vi "Host Image Acquisition Module.vi"(0 "Operation":T3=enum."Close FPGA", 11 "error in":errorcluster={"status"=FALSE, "code"=61003, "source"="niLvFpga_Run_PCIe-1473R-LX110.vi"}) -> (1 "Number of Elements to Read Cam Data":u32, 3 "Num Frames read":u32, 4 "Image":T2(plugin-control), 6 "Acq In Progress":bool, 8 "error out":errorcluster={"status"=FALSE, "code"=61003, "source"="niLvFpga_Run_PCIe-1473R-LX110.vi"}, 10 "Image Acquired":bool, 12 "Number of Elements to Write Host DMA":u32, 14 "DMA Write Timeout":bool, 15 "Frames To Acquire":u32=1)   [LabVIEW 2013]
uses:
  Host Image Acquisition Module Enum.ctl
  Acquisition Settings Cluster.ctl
  Image Acquisition Settings FG Enum.ctl
  Common/CL Configuration.ctl
  Common/CL Signal Mapping.ctl
  System Status/Status FG Enum.ctl
  Image Processing/Mask ROI FG Enum.ctl
  <vilib>/rvi/interface/common/niFpgaWaitOnOcc.vi
  Globals/Average Sector Data.vi
  <vilib>/Utility/error.llb/Error Cluster From Error Code.vi
  <vilib>/rvi/errors/niLvFpgaAdjustHostInterfaceError.vi
  <vilib>/FPGAPlugInAG/PCIe-1473R-LX110/niLvFpga_Run_PCIe-1473R-LX110.vi
  <vilib>/FPGAPlugInAG/PCIe-1473R-LX110/niLvFpga_Close_PCIe-1473R-LX110.vi
  <vilib>/rvi/interface/nirviReadWriteControl/nirviReadWriteControl.xnode
  FGs/FPGA_Reference.ctl
  FPGA Bitfiles/WBA256SectorsSim_FPGATarget.lvbitx
  <vilib>/rvi/interface/nirviMethod/nirviMethod.xnode
  FPGA/Sector/Accumulate/Sector Parameter Cluster.ctl
  <vilib>/rvi/interface/nirviCloseFPGA/nirviCloseFPGA.xnode
  Common/Timing/Timing Lib.lvlib
  NiFpgaLv.dll
  <vilib>/FPGAPlugInAG/PCIe-1473R-LX110/niLvFpga_ReadFifo_PCIe-1473R-LX110.vi
  <vilib>/rvi/errors/niLvFpgaMergeErrorWithErrorCode.vi
  <vilib>/FPGAPlugInAG/PCIe-1473R-LX110/niLvFpga_ConfigureFifo_PCIe-1473R-LX110.vi
  <vilib>/FPGAPlugInAG/PCIe-1473R-LX110/niLvFpga_StartFifo_PCIe-1473R-LX110.vi
  <vilib>/FPGAPlugInAG/PCIe-1473R-LX110/niLvFpga_Reset_PCIe-1473R-LX110.vi
panel:
  out "Actual Depth":u32=53190144
  out "Target Sim TO":bool
  out "Cam Data Timeout":bool
  out "Sector FIFO Timeout":bool
  out "Host DMA Timeout":bool
  out "Elements Remaining":u32
  out "Words per image":u32=118200
  out "DMA Words per Image":u32=118200
  out "Acquire":bool=TRUE
  in  "Acquisition Settings Cluster":T1={"Image Width"=1200, "Image Height"=788, "Frames To Acquire"=0, "Signal Mapping"=enum."Basler 10-tap", "DMA Buffer Size\n(In Images)"=64} {"Image Height" max=65535; "Image Width" max=65535 step=40}
  out "Buffer Size":u32=53190000
  out "Acq'd Frame Width":u32
  in  "Start Serial Server":bool
  out "Frames Acq'd":u32=1
  out "Acq'd Frame Height":u32
  out "Initialized":bool
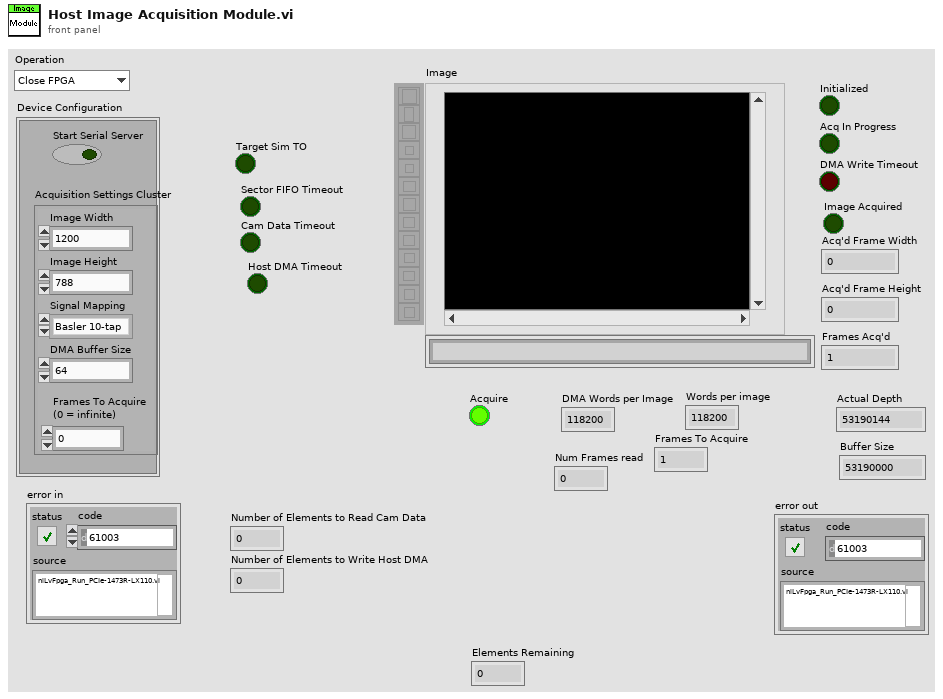
[diagram p1: front panel]
types:
  T1 = typedef "Acquisition Settings Cluster.ctl" = cluster{"Image Width":u32, "Image Height":u32, "Frames To Acquire":u32, "Signal Mapping":enum8{"Standard", "Basler 10-tap", "Vosskühler 10-tap"}, "DMA Buffer Size\n(In Images)":u32}
  T2 = typedef "IMAQ Image.ctl" = refnum<image>
  T3 = typedef "Host Image Acquisition Module Enum.ctl" = enum16{"Open FPGA", "Initialize DMA FIFO", "Load Sim Images", "Initialize Acquisition", "Update Sector Parameters", "Start Acquisition", "Aquire Image", "Read Averages", "Cancel Acquisition", "Close FPGA"}
  T4 = typedef "CL Signal Mapping.ctl" = enum8{"Standard", "Basler 10-tap", "Vosskühler 10-tap"}
  T5 = typedef "CL Configuration.ctl" = enum8{"Base", "Medium", "Full"}
  T6 = typedef "Image Acquisition Settings FG Enum.ctl" = enum16{"Read", "Write"}
  T7 = typedef "Status FG Enum.ctl" = enum16{"Reset", "Read", "Write"}
  T8 = typedef "Mask ROI FG Enum.ctl" = enum16{"Read", "Write", "Enable Background", "Disable Background"}
  T9 = enum16{"big-endian, network order", "native, host order", "little-endian"}
  T10 = typedef "FPGA_Reference.ctl" = refnum<k20>
  T11 = typedef "Mask ROI Cluster.ctl" = cluster{"left annulus":T12, "right annulus":T12, "Threshold Range":cluster{"Lower value":dbl, "Upper value":dbl}, "[Avg BG]":u8[], "Number of Sectors":u8, "Left ROI":T13, "Right ROI":T13, "Left Start Angle Duty Cycle":fxp<+,8,0>, "Left End Angle Duty Cycle":fxp<+,8,0>, "Right End Angle Duty Cycle":fxp<+,8,0>, "Right Start Angle Duty Cycle":fxp<+,8,0>, "[Sector ROIs]":T13[]}
  T12 = typedef "IMAQ Circle" = cluster{"Center X":i32, "Center Y":i32, "Inner Radius":i32, "Outer Radius":i32, "Start Angle":dbl, "End Angle":dbl}
  T13 = typedef "ROI Descriptor" = cluster{"Global Rectangle":i32[], "Contours":cluster{"ID":enum32{"External", "Internal"}, "Type":u32, "Coordinates":i32[]}[]}
  T14 = typedef "Sector Parameter Cluster.ctl" = cluster{"Start Angle":fxp<+/-,17,2>, "End Angle":fxp<+/-,17,2>, "Inner Radius":u16, "Outter Radius":u16, "Hinge X":u16, "Hinge Y":u16, "NumWingSectors":u8}
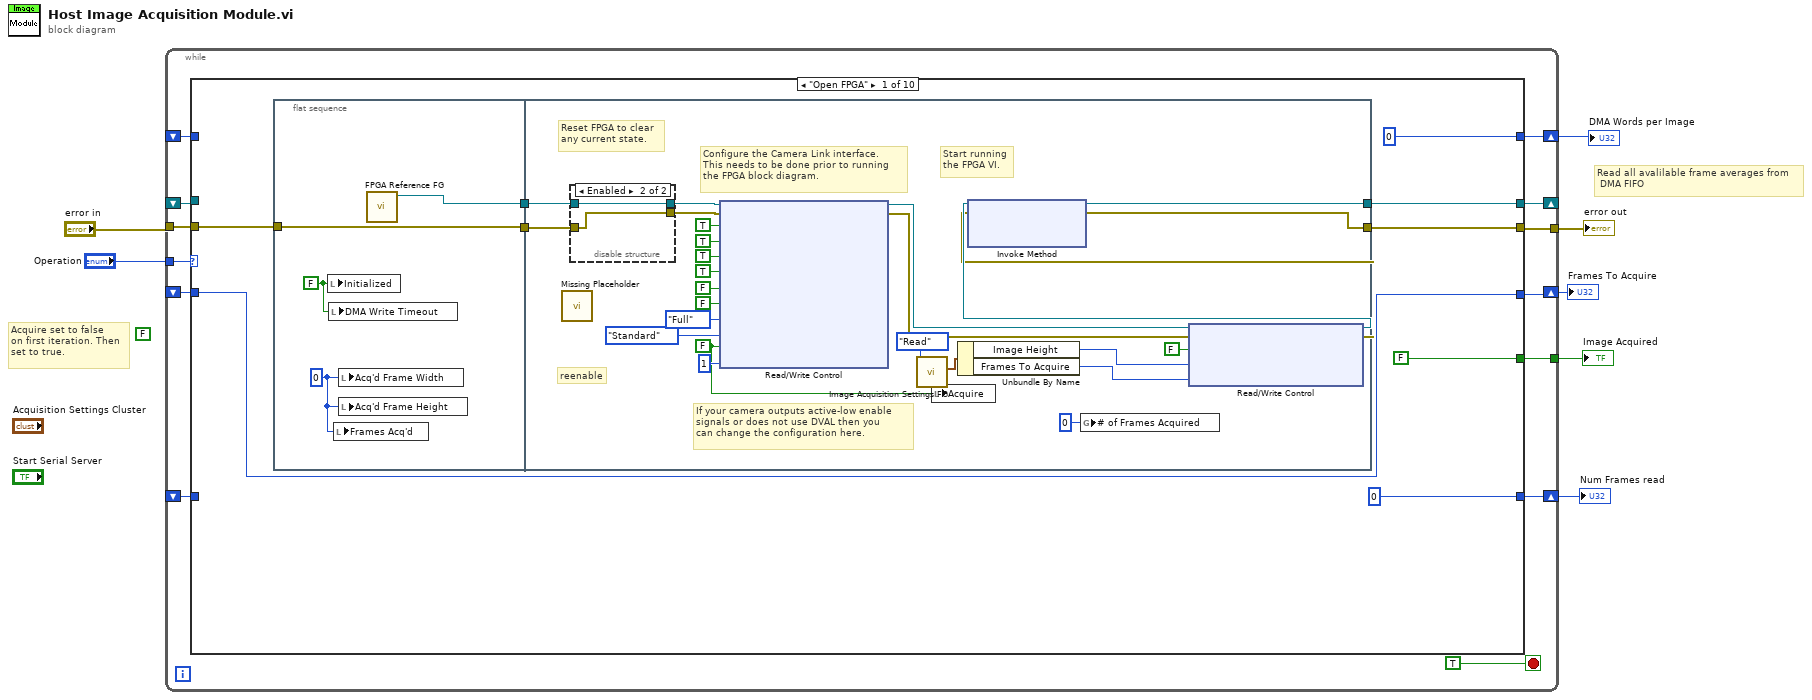
[diagram p0: block diagram]
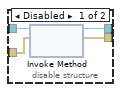
[diagram p2: hidden frame]
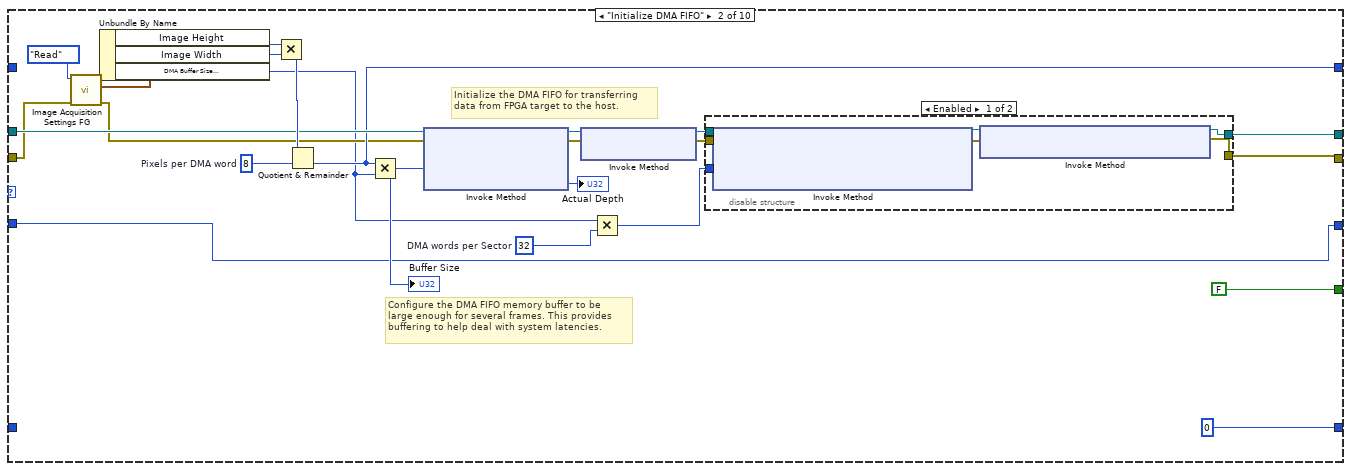
[diagram p3: hidden frame]
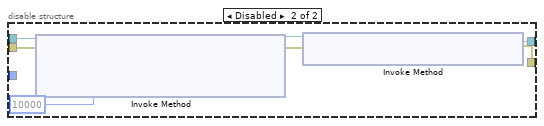
[diagram p4: hidden frame]
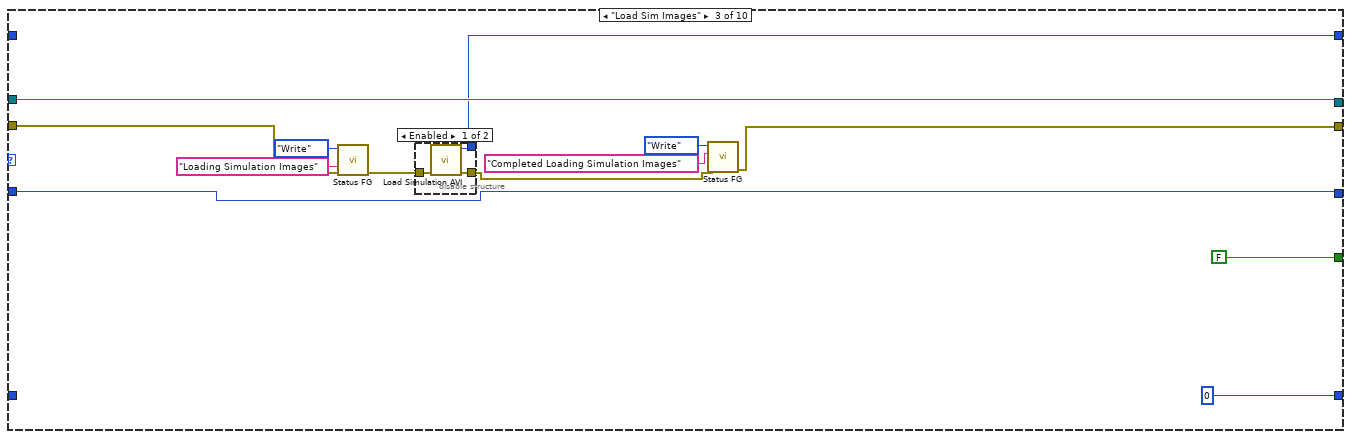
[diagram p5: hidden frame]
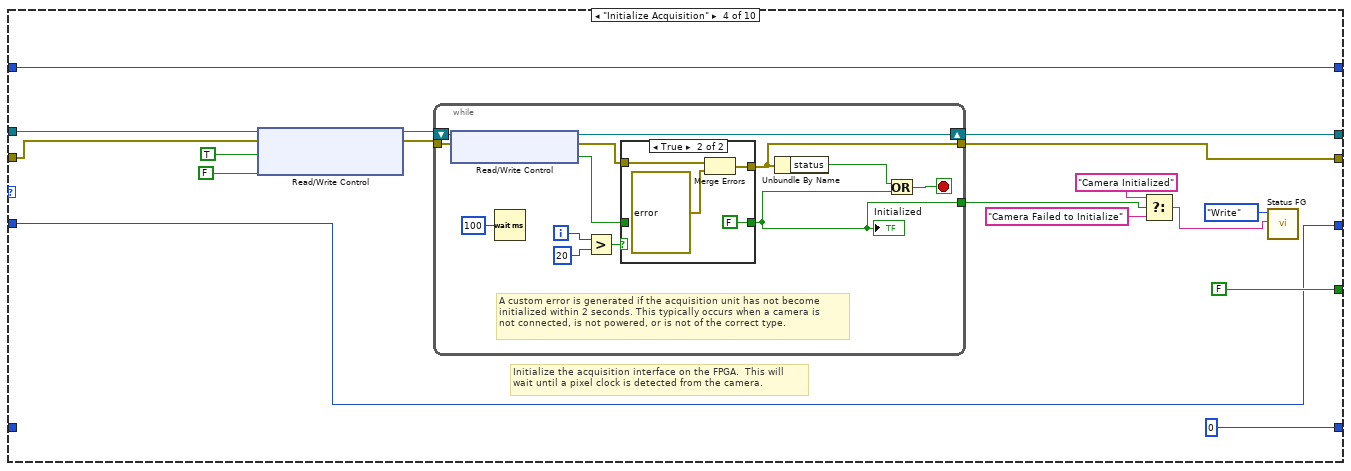
[diagram p7: hidden frame]
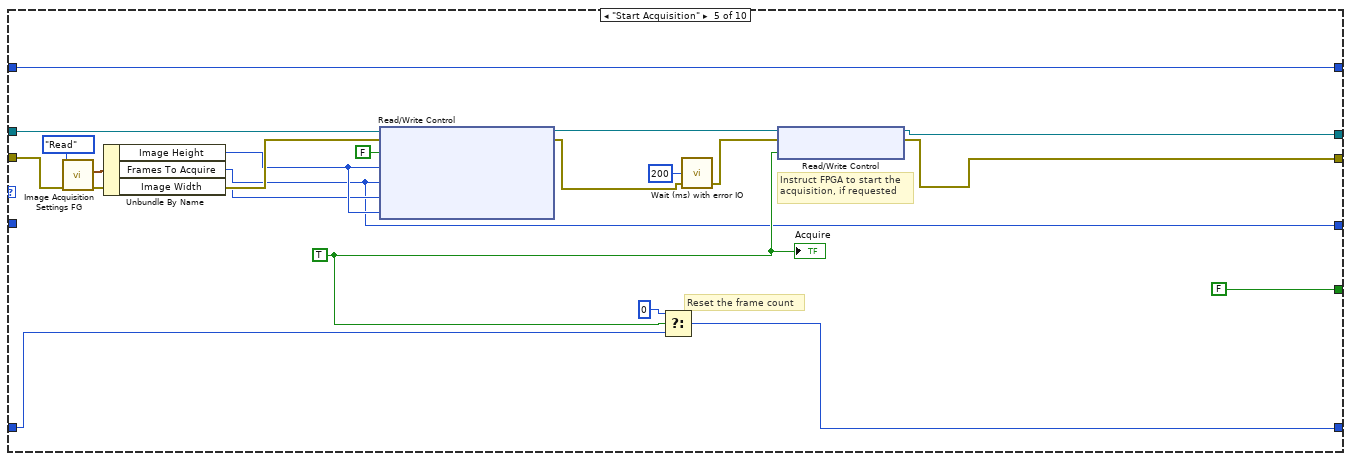
[diagram p9: hidden frame]
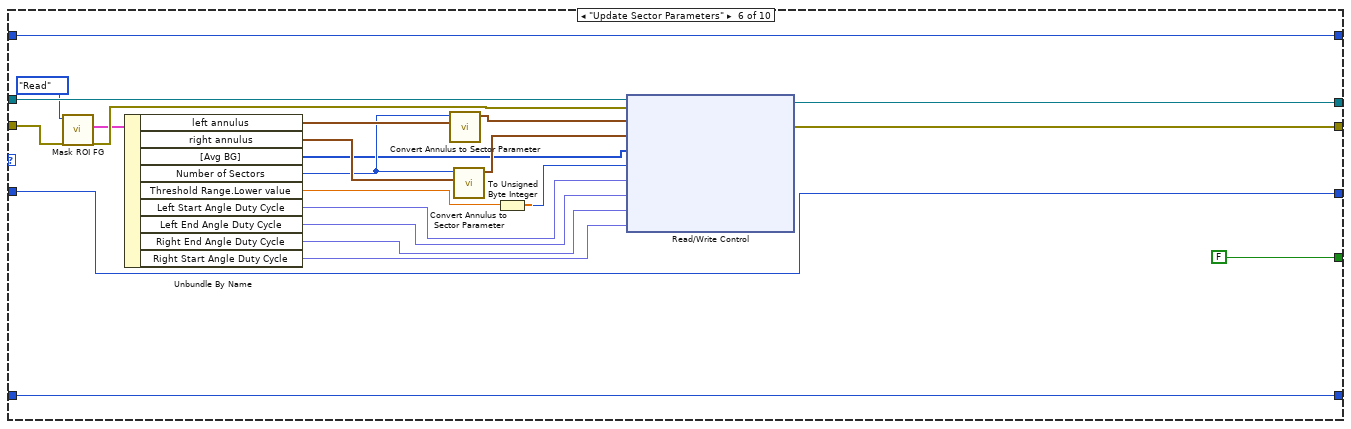
[diagram p10: hidden frame]
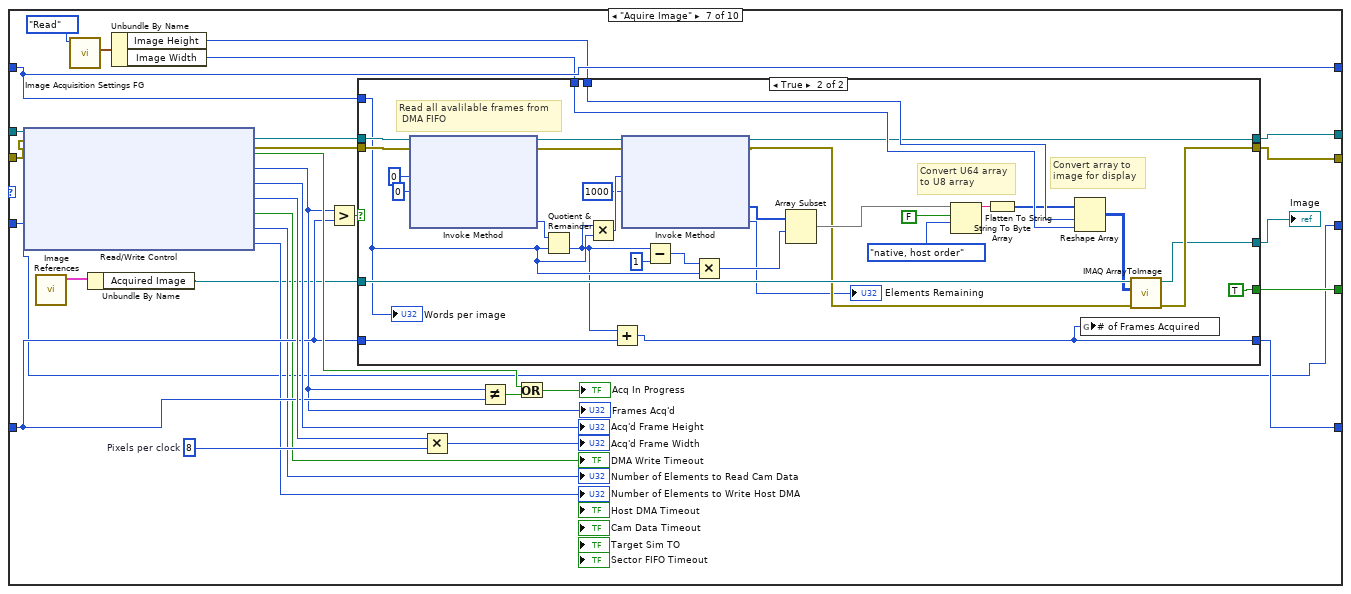
[diagram p11: hidden frame]
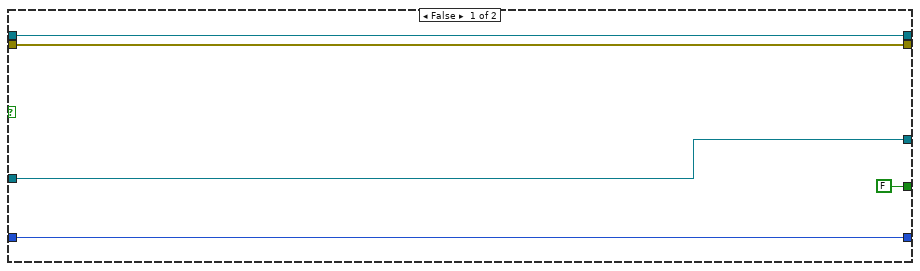
[diagram p12: hidden frame]
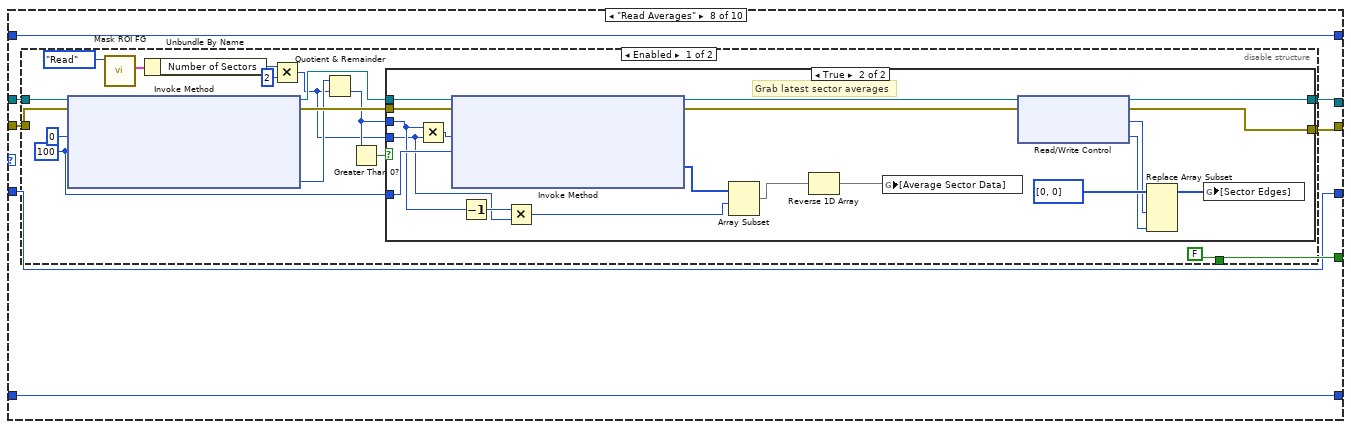
[diagram p13: hidden frame]
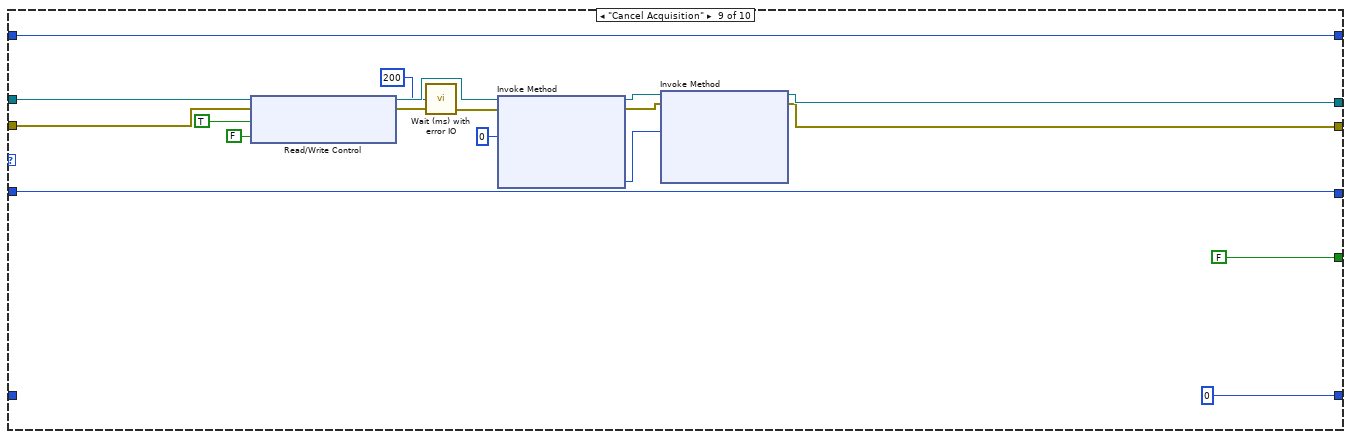
[diagram p16: hidden frame]
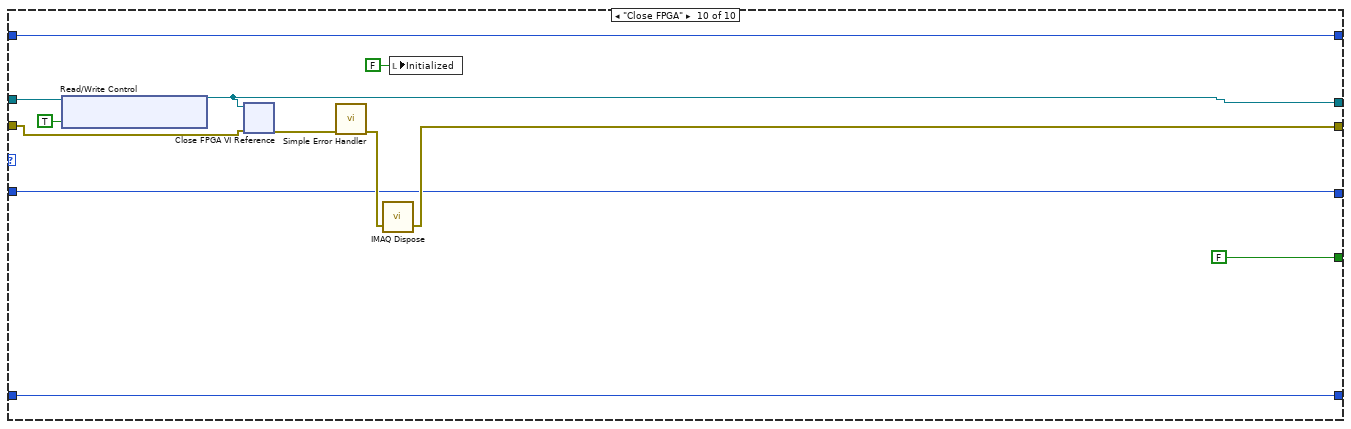
[diagram p17: hidden frame]
diagram:
  (unwired) FALSE ("Acquire")
  # "Read all avalilable frame averages from\n DMA FIFO"
  # "Acquire set to false\non first iteration. Then\nset to true."
  n1 = while {
    shift-right: [w19] -> _
    shift-left: _ -> [w15]
    tunnel: "error in" -> [w18]
    tunnel: "Operation" -> [w17]
    tunnel: [w16] -> w5
    shift-right: [w14] -> w4
    shift-left: _ -> [w13]
    shift-right: [w12] -> w3
    shift-left: _ -> [w11]
    tunnel: [w10] -> w2
    shift-right: [w9] -> w1
    shift-left: _ -> [w8]
    stop <- TRUE stop-if-true
    n2 = case shown="\"Open FPGA\"" w17 {
      tunnel: w18 -> [w29 w79 w112 w128 w172 w198 w214 w269 w331 w336]
      tunnel: [w28 w75 w115 w133 w166 w194 w229 w274 w317 w337] -> w19
      tunnel: [w27 w70 w106 w129 w165 w195 w228 w270 w316 w342] -> w16
      tunnel: w15 -> [_ w84 w115 w134 w173 w200 w230 w275 w333 w339]
      tunnel: [u32 0 w83 w114 w132 w168 w199 w223 w273 w330 w340] -> w14
      tunnel: w13 -> [_ _ _ w132 w168 w199 w223 w273 w330 w340]
      tunnel: [u32 0 u32 0 u32 0 u32 0 w169 w193 w227 w272 u32 0 w341] -> w12
      tunnel: w11 -> [_ _ _ _ w170 w193 w212 w272 _ w341]
      tunnel: [FALSE ("Image Acquired") FALSE ("Image Acquired") FALSE ("Image Acquired") FALSE ("Image Acquired") FALSE ("Image Acquired") FALSE ("Image Acquired") w208 w271 FALSE ("Image Acquired") FALSE ("Image Acquired")] -> w10
      tunnel: [w21 w66 w104 w121 w157 w178 w201 w268 w326 w334] -> w9
      tunnel: w8 -> [w21 w66 w104 w121 _ w178 w201 w268 w326 w334]
      frame "Open FPGA" {
        n3 = flat-sequence {
          tunnel: w29 -> [w30]
          tunnel: [w31] -> w26
          tunnel: [w30] -> w25
          tunnel: [w48] -> w27
          tunnel: [w49] -> w28
          tunnel: w26 -> [w52]
          tunnel: w25 -> [w50]
          frame #0 {
            w32 = u32 0 ("Acq'd Frame Width")
            w33 = FALSE ("Initialized")
            n4 = local write "Initialized"(w33) -> ()
            n5 = local write "DMA Write Timeout"(w33) -> ()
            n6 = local write "Frames Acq'd"(w32) -> ()
            n7 = local write "Acq'd Frame Width"(w32) -> ()
            n8 = local write "Acq'd Frame Height"(w32) -> ()
            n9 = call "FPGA Reference FG.vi"() -> ("FPGA VI Reference Out"=w31:T10)  [unwired: 11 in]
          }
          frame #1 {
            w46 = FALSE ("Acq Control.Acquire")
            # "reenable"
            # "If your camera outputs active-low enable\nsignals or does not use DVAL then you \ncan change the configuration here."
            # "Start running\nthe FPGA VI."
            # "Reset FPGA to clear\nany current state."
            # "Configure the Camera Link interface.\nThis needs to be done prior to running\nthe FPGA block diagram."
            n10 = call "Missing Placeholder.vi"() -> ()  [unwired: 12 in]
            n11 = disable-structure shown="Enabled" {
              disable-tunnel: [w63 w65] -> w54
              disable-tunnel: [w62 w64] -> w53
              disable-tunnel: w52 -> [w61 w65]
              disable-tunnel: w50 -> [w60 w64]
              frame Disabled {
                n12 = xnode "Invoke Method"("FPGA VI Reference In"=w61, "error in"=w60) -> ("FPGA VI Reference Out"=w63:T10, "error out"=w62:errorcluster)
              }
              frame Enabled {
              }
            }
            n13 = xnode "Read/Write Control"("FPGA VI Reference In"=w54, "error in"=w53, "CL Config.FVAL Active High"=TRUE ("IO Module Config.CL FVAL Active High"), "CL Config.LVAL Active High"=TRUE ("IO Module Config.CL LVAL Active High"), "CL Config.DVAL Active High"=TRUE ("IO Module Config.CL DVAL Active High"), "CL Config.Spare Active High"=TRUE ("IO Module Config.CL Spare Active High"), "CL Config.Line Scan"=FALSE, "Acq Control.Ignore DVAL"=FALSE ("CL Config.Line Scan"), "CL Config.Configuration"=CL_Configuration."Full", "CL Config.Signal Mapping"=CL_Signal_Mapping."Standard", "Acq Control.Acquire"=w46, "# of Frames to Average"=u8 1) -> ("FPGA VI Reference Out"=w41:T10, "error out"=w39:errorcluster)
            n14 = call "Image Acquisition Settings FG.vi"("Operation"=Image_Acquisition_Settings_FG_Enum."Read") -> ("Acquisition Settings Out"=w45:T1)  [unwired: 9 in, 1 out]
            n15 = local write "Acquire"(w46) -> ()
            n16 = Unbundle By Name(w45) -> ("Image Height"=w43:u32, "Frames To Acquire"=w37:u32)
            n17 = global write "Average Sector Data.vi" "# of Frames Acquired"(u32 0 ("# of Frames Acquired")) -> ()
            n18 = xnode "Read/Write Control"("FPGA VI Reference In"=w41, "error in"=w39, "Acq Control.Cancel Acq"=FALSE, "Acq Control.Line Scan Height"=w43, "Acq Control.Frames To Acq"=w37) -> ("FPGA VI Reference Out"=w40:T10, "error out"=w38:errorcluster)
            n19 = xnode "Invoke Method"("FPGA VI Reference In"=w40, "error in"=w38) -> ("FPGA VI Reference Out"=w49:T10, "error out"=w48:errorcluster)  [unwired: 1 in]
          }
        }
      }
      frame "Initialize DMA FIFO" {
        w69 = u32 32  # DMA words per Sector
        w86 = u32 8  # Pixels per DMA word
        # "Configure the DMA FIFO memory buffer to be\nlarge enough for several frames. This provides\nbuffering to help deal with system latencies."
        # "Initialize the DMA FIFO for transferring\ndata from FPGA target to the host."
        n20 = call "Image Acquisition Settings FG.vi"("error in (no error)"=w79, "Operation"=Image_Acquisition_Settings_FG_Enum."Read") -> ("error out"=w76:errorcluster, "Acquisition Settings Out"=w80:T1)  [unwired: 8 in]
        n21 = Unbundle By Name(w80) -> ("Image Height"=w78:u32, "Image Width"=w77:u32, "DMA Buffer Size\n(In Images)"=w68:u32)
        n22 = Multiply(x=w78, y=w77) -> (x*y=w85:u32)
        n23 = Quotient & Remainder(x=w85, y=w86) -> (floor(x/y)=w83:u32)  [unwired: 1 out]
        n24 = Multiply(x=w83, y=w68) -> (x*y=w87:u32)
        "Buffer Size" <- w87
        n25 = xnode "Invoke Method"("FPGA VI Reference In"=w84, "error in"=w76, "Requested Depth"=w87) -> ("FPGA VI Reference Out"=w89:T10, "error out"=w88:errorcluster, "Actual Depth"=→"Actual Depth":u32)
        n26 = xnode "Invoke Method"("FPGA VI Reference In"=w89, "error in"=w88) -> ("FPGA VI Reference Out"=w73:T10, "error out"=w71:errorcluster)
        n27 = Multiply(x=w68, y=w69) -> (x*y=w67:u32)
        n28 = disable-structure shown="Enabled" {
          disable-tunnel: w67 -> [w96 _]
          disable-tunnel: [w95 w103] -> w75
          disable-tunnel: w73 -> [w94 w102]
          disable-tunnel: w71 -> [w93 w101]
          disable-tunnel: [w90 w98] -> w70
          frame Enabled {
            n29 = xnode "Invoke Method"("FPGA VI Reference In"=w94, "error in"=w93, "Requested Depth"=w96) -> ("FPGA VI Reference Out"=w92:T10, "error out"=w91:errorcluster)  [unwired: 1 out]
            n30 = xnode "Invoke Method"("FPGA VI Reference In"=w92, "error in"=w91) -> ("FPGA VI Reference Out"=w95:T10, "error out"=w90:errorcluster)
          }
          frame Disabled {
            n31 = xnode "Invoke Method"("FPGA VI Reference In"=w102, "error in"=w101, "Requested Depth"=u32 10000) -> ("FPGA VI Reference Out"=w100:T10, "error out"=w99:errorcluster)  [unwired: 1 out]
            n32 = xnode "Invoke Method"("FPGA VI Reference In"=w100, "error in"=w99) -> ("FPGA VI Reference Out"=w103:T10, "error out"=w98:errorcluster)
          }
        }
      }
      frame "Load Sim Images" {
        n33 = call "Status FG.vi"("error in (no error)"=w112, "Status In"="Loading Simulation Images", "Operation"=Status_FG_Enum."Write") -> ("error out"=w111:errorcluster)  [unwired: 7 in, 1 out]
        n34 = disable-structure shown="Enabled" {
          disable-tunnel: [w119 _] -> w114
          disable-tunnel: w111 -> [w118 w120]
          disable-tunnel: [w117 w120] -> w107
          frame Enabled {
            n35 = call "Load Simulation AVI.vi"("error in (no error)"=w118) -> ("error out"=w117:errorcluster, "Words per image"=w119:u32)  [unwired: 9 in]
          }
          frame Disabled {
          }
        }
        n36 = call "Status FG.vi"("error in (no error)"=w107, "Status In"="Completed Loading Simulation Images", "Operation"=Status_FG_Enum."Write") -> ("error out"=w106:errorcluster)  [unwired: 7 in, 1 out]
      }
      frame "Initialize Acquisition" {
        # "Initialize the acquisition interface on the FPGA.  This will\nwait until a pixel clock is detected from the camera."
        n37 = xnode "Read/Write Control"("FPGA VI Reference In"=w134, "error in"=w128, "Acq Control.Initialize"=TRUE ("Arm Acquisition"), "Acq Control.Cancel Acq"=FALSE) -> ("FPGA VI Reference Out"=w137:T10, "error out"=w136:errorcluster)
        n38 = while {
          tunnel: w136 -> [w145]
          tunnel: [w147] -> w129
          shift-right: [w144] -> w133
          shift-left: w137 -> [w146]
          tunnel: [w138] -> w124
          i -> [w140]
          stop <- w150 stop-if-true
          # "A custom error is generated if the acquisition unit has not become\ninitialized within 2 seconds. This typically occurs when a camera is\nnot connected, is not powered, or is not of the correct type."
          n39 = xnode "Read/Write Control"("FPGA VI Reference In"=w146, "error in"=w145) -> ("FPGA VI Reference Out"=w144:T10, "error out"=w143:errorcluster, "Acq Status.Initialized"=w142:bool)
          n40 = Wait (ms)(milliseconds to wait=u32 100) -> ()  [unwired: 1 out]
          n41 = Greater?(x=w140, y=20) -> (0:w141:bool)
          n42 = case shown="True" w141 {
            tunnel: [w152 FALSE] -> w138
            tunnel: w142 -> [w152 _]
            tunnel: w143 -> [w151 w154]
            tunnel: [w151 w156] -> w147
            frame False {
            }
            frame True {
              n43 = Merge Errors(w154, errorcluster {"status"=TRUE, "code"=-8999, "source"="Acquisition Initialization: This error typically occurs when a camera is not properly connected, is not powered, or is not of the correct type."} ("error in")) -> (w156:errorcluster)
            }
          }
          "Initialized" <- w138
          n44 = Unbundle By Name(w147) -> ("status"=w149:bool)
          n45 = Or(x=w149, y=w138) -> (x .or. y?=w150:bool)
        }
        n46 = Select(t="Camera Initialized", s=w124, f="Camera Failed to Initialize") -> (s? t:f=w126:string)
        n47 = call "Status FG.vi"("Status In"=w126, "Operation"=Status_FG_Enum."Write") -> ()  [unwired: 8 in, 2 out]
      }
      frame "Start Acquisition" {
        w174 = TRUE ("Acquire")
        # "Reset the frame count"
        # "Instruct FPGA to start the\nacquisition, if requested"
        n48 = call "Image Acquisition Settings FG.vi"("error in (no error)"=w172, "Operation"=Image_Acquisition_Settings_FG_Enum."Read") -> ("error out"=w171:errorcluster, "Acquisition Settings Out"=w177:T1)  [unwired: 8 in]
        n49 = Unbundle By Name(w177) -> ("Image Height"=w159:u32, "Frames To Acquire"=w157:u32, "Image Width"=w158:u32)
        n50 = xnode "Read/Write Control"("FPGA VI Reference In"=w173, "error in"=w171, "Acq Control.Cancel Acq"=FALSE, "Acq Control.Line Scan Height"=w159, "Acq Control.Frames To Acq"=w157, "X Resolution"=w158, "Y Resolution"=w159) -> ("FPGA VI Reference Out"=w163:T10, "error out"=w162:errorcluster)
        n51 = Select(t=u32 0, s=w174, f=w170) -> (s? t:f=w169:u32)
        n52 = call "Wait (ms) with error IO.vi"("error in (no error)"=w162, "milliseconds to wait"=u32 200) -> ("error out"=w161:errorcluster)  [unwired: 3 in]
        n53 = xnode "Read/Write Control"("FPGA VI Reference In"=w163, "error in"=w161, "Acq Control.Acquire"=w174) -> ("FPGA VI Reference Out"=w166:T10, "error out"=w165:errorcluster)
        "Acquire" <- w174
      }
      frame "Update Sector Parameters" {
        n54 = call "Mask ROI FG.vi"("error in (no error)"=w198, "Operation"=Mask_ROI_FG_Enum."Read") -> ("error out"=w197:errorcluster, "Mask ROI Out"=w192:T11)  [unwired: 8 in]
        n55 = Unbundle By Name(w192) -> ("left annulus"=w191:T12, "right annulus"=w189:T12, "[Avg BG]"=w186:u8[], "Number of Sectors"=w188:u8, "Threshold Range.Lower value"=w184:dbl, "Left Start Angle Duty Cycle"=w182:fxp<+,8,0>, "Left End Angle Duty Cycle"=w181:fxp<+,8,0>, "Right End Angle Duty Cycle"=w180:fxp<+,8,0>, "Right Start Angle Duty Cycle"=w179:fxp<+,8,0>)
        n56 = call "Convert Annulus to Sector Parameter.vi"("Annulus"=w191, "NumWingSectors"=w188) -> ("Sector Parameter"=w190:T14)  [unwired: 9 in]
        n57 = call "Convert Annulus to Sector Parameter.vi"("Annulus"=w189, "NumWingSectors"=w188) -> ("Sector Parameter"=w187:T14)  [unwired: 9 in]
        n58 = To Unsigned Byte Integer(number=w184) -> (unsigned 8bit integer=w183:u8)
        n59 = xnode "Read/Write Control"("FPGA VI Reference In"=w200, "error in"=w197, "Sector Parameters Left"=w190, "Sector Parameters Right"=w187, "[Average BG Intensity]"=w186, "Sector Threshold"=w183, "Left Start Angle Duty Cycle"=w182, "Left End Angle Duty Cycle"=w181, "Right End Angle Duty Cycle"=w180, "Right Start Angle Duty Cycle"=w179) -> ("FPGA VI Reference Out"=w194:T10, "error out"=w195:errorcluster)
      }
      frame "Aquire Image" {
        w221 = u32 8  # Pixels per clock
        n60 = xnode "Read/Write Control"("FPGA VI Reference In"=w230, "error in"=w214) -> ("FPGA VI Reference Out"=w226:T10, "error out"=w225:errorcluster, "Acq Status.Acq In Progress"=w213:bool, "Acq Status.Frames Acq'd"=w211:u32, "Acq Status.Lines Per Frame"=→"Acq'd Frame Height":u32, "Acq Status.Clocks Per Line"=w220:u32, "Acq Status.DMA Write Timeout"=→"DMA Write Timeout":bool, "Number of Elements to Read Cam Data"=→"Number of Elements to Read Cam Data":u32, "Number of Elements to Write Host DMA"=→"Number of Elements to Write Host DMA":u32)
        "Frames Acq'd" <- w211
        n61 = call "Image References.vi"() -> ("Images"=w204:cluster{"Acquired Image":T2, "Display Image":T2})  [unwired: 10 in, 1 out]
        n62 = call "Image Acquisition Settings FG.vi"("Operation"=Image_Acquisition_Settings_FG_Enum."Read") -> ("Acquisition Settings Out"=w217:T1)  [unwired: 9 in, 1 out]
        n63 = Unbundle By Name(w204) -> ("Acquired Image"=w203:T2)
        n64 = Unbundle By Name(w217) -> ("Image Height"=w216:u32, "Image Width"=w215:u32)
        n65 = Greater?(x=w211, y=w212) -> (0:w224:bool)
        n66 = case shown="True" w224 {
          tunnel: w226 -> [w234 w259]
          tunnel: w225 -> [w233 w260]
          tunnel: w216 -> [_ w267]
          tunnel: w215 -> [_ w266]
          tunnel: w203 -> [w235 w265]
          tunnel: [w233 w264] -> w228
          tunnel: [w234 w240] -> w229
          tunnel: w212 -> [w232 w263]
          tunnel: [w232 w238] -> w227
          tunnel: w223 -> [_ w245]
          tunnel: [w235 w262] -> w202
          tunnel: [FALSE ("Image Acquired") TRUE ("Image Acquired")] -> w208
          frame False {
          }
          frame True {
            # "Convert U64 array\nto U8 array"
            # "Convert array to\nimage for display"
            # "Read all avalilable frames from\n DMA FIFO"
            n67 = xnode "Invoke Method"("FPGA VI Reference In"=w259, "error in"=w260, "Number of Elements"=u32 0, "Timeout (ms)"=0) -> ("FPGA VI Reference Out"=w256:T10, "error out"=w255:errorcluster, "Elements Remaining"=w254:u32)  [unwired: 1 out]
            n68 = Quotient & Remainder(x=w254, y=w245) -> (floor(x/y)=w236:u32)  [unwired: 1 out]
            n69 = Multiply(x=w236, y=w245) -> (x*y=w253:u32)
            n70 = Add(x=w236, y=w263) -> (x+y=w238:u32)
            n71 = xnode "Invoke Method"("FPGA VI Reference In"=w256, "error in"=w255, "Number of Elements"=w253, "Timeout (ms)"=1000) -> ("FPGA VI Reference Out"=w240:T10, "error out"=w241:errorcluster, "Data"=w244:u64[], "Elements Remaining"=→"Elements Remaining":u32)
            n72 = Subtract(x=w236, y=u32 1) -> (x-y=w246:u32)
            n73 = Multiply(x=w246, y=w245) -> (x*y=w243:u32)
            n74 = Array Subset(array=w244, index=w243) -> (w242:u64[])  [unwired: 1 in]
            n75 = Flatten To String(anything=w242, prepend array or string size? (T)=FALSE, byte order (0:big-endian, network order)=T9."native, host order") -> (data string=w248:string)  [unwired: 1 in, 2 out]
            n76 = String To Byte Array(string=w248) -> (unsigned byte array=w247:u8[])
            n77 = Reshape Array(w247, w267, w266) -> (w251:u8[][])
            n78 = global write "Average Sector Data.vi" "# of Frames Acquired"(w238) -> ()
            n79 = call "IMAQ ArrayToImage"("error in (no error)"=w241, "Image Pixels (U8)"=w251, "Image"=w265) -> ("error out"=w264:errorcluster, "Image Out"=w262:T2)  [unwired: 7 in]
            "Words per image" <- w245
          }
        }
        "Image" <- w202
        n80 = Multiply(x=w220, y=w221) -> (x*y=→"Acq'd Frame Width":u32)
        n81 = Not Equal?(x=w211, y=w212) -> (x != y?=w210:bool)
        n82 = Or(x=w213, y=w210) -> (x .or. y?=→"Acq In Progress":bool)
      }
      frame "Read Averages" {
        n83 = disable-structure shown="Enabled" {
          disable-tunnel: w275 -> [w292 w315]
          disable-tunnel: [w291 w315] -> w274
          disable-tunnel: [FALSE ("Image Acquired") _] -> w271
          disable-tunnel: [w289 w314] -> w270
          disable-tunnel: w269 -> [w288 w314]
          frame Enabled {
            w284 = 100 ("Timeout (ms)")
            n84 = xnode "Invoke Method"("FPGA VI Reference In"=w292, "error in"=w288, "Number of Elements"=u32 0, "Timeout (ms)"=w284) -> ("FPGA VI Reference Out"=w286:T10, "error out"=w285:errorcluster, "Elements Remaining"=w279:u32)  [unwired: 1 out]
            n85 = call "Mask ROI FG.vi"("Operation"=Mask_ROI_FG_Enum."Read") -> ("Mask ROI Out"=w282:T11)  [unwired: 9 in, 1 out]
            n86 = Unbundle By Name(w282) -> ("Number of Sectors"=w281:u8)
            n87 = Multiply(x=w281, y=u8 2) -> (x*y=w276:u8)
            n88 = Quotient & Remainder(x=w279, y=w276) -> (floor(x/y)=w277:u32)  [unwired: 1 out]
            n89 = Greater Than 0?(x=w277) -> (x > 0?=w278:bool)
            n90 = case shown="True" w278 {
              tunnel: w286 -> [w294 w313]
              tunnel: w285 -> [w293 w312]
              tunnel: w284 -> [_ w311]
              tunnel: [w294 w307] -> w291
              tunnel: [w293 w308] -> w289
              tunnel: w277 -> [_ w299]
              tunnel: w276 -> [_ w298]
              frame False {
              }
              frame True {
                # "Grab latest sector averages"
                n91 = Multiply(x=w299, y=w298) -> (x*y=w301:u32)
                n92 = xnode "Invoke Method"("FPGA VI Reference In"=w313, "error in"=w312, "Number of Elements"=w301, "Timeout (ms)"=w311) -> ("FPGA VI Reference Out"=w310:T10, "error out"=w309:errorcluster, "Data"=w297:u8[])  [unwired: 1 out]
                n93 = Decrement(x=w299) -> (x-1=w300:u32)
                n94 = Multiply(x=w300, y=w298) -> (x*y=w296:u32)
                n95 = Array Subset(array=w297, index=w296) -> (w295:u8[])  [unwired: 1 in]
                n96 = Reverse 1D Array(array=w295) -> (reversed array=w306:u8[])
                n97 = global write "Average Sector Data.vi" "[Average Sector Data]"(w306) -> ()
                n98 = xnode "Read/Write Control"("FPGA VI Reference In"=w310, "error in"=w309) -> ("FPGA VI Reference Out"=w307:T10, "error out"=w308:errorcluster, "Right Sector Edge"=w304:u16, "Left Sector Edge"=w303:u16)
                n99 = Replace Array Subset(array=u8[] [0, 0] ("[Sector Edges]"), new element #1=w304, new element #2=w303) -> (w302:u8[])  [unwired: 2 in]
                n100 = global write "Average Sector Data.vi" "[Sector Edges]"(w302) -> ()
              }
            }
          }
          frame Disabled {
          }
        }
      }
      frame "Cancel Acquisition" {
        n101 = xnode "Read/Write Control"("FPGA VI Reference In"=w333, "error in"=w331, "Acq Control.Cancel Acq"=TRUE, "Acq Control.Acquire"=FALSE) -> ("FPGA VI Reference Out"=w319:T10, "error out"=w321:errorcluster)
        n102 = call "Wait (ms) with error IO.vi"("error in (no error)"=w321, "milliseconds to wait"=u32 200) -> ("error out"=w320:errorcluster)  [unwired: 3 in]
        n103 = xnode "Invoke Method"("FPGA VI Reference In"=w319, "error in"=w320, "Number of Elements"=u32 0) -> ("FPGA VI Reference Out"=w324:T10, "error out"=w323:errorcluster, "Elements Remaining"=w322:u32)  [unwired: 1 in, 1 out]
        n104 = xnode "Invoke Method"("FPGA VI Reference In"=w324, "error in"=w323, "Number of Elements"=w322) -> ("FPGA VI Reference Out"=w317:T10, "error out"=w316:errorcluster)  [unwired: 1 in, 2 out]
      }
      frame "Close FPGA" {
        n105 = xnode "Read/Write Control"("FPGA VI Reference In"=w339, "Acq Control.Cancel Acq"=TRUE) -> ("FPGA VI Reference Out"=w337:T10)  [unwired: 1 in, 1 out]
        n106 = xnode "Close FPGA VI Reference"("FPGA VI Reference In"=w337, "error in"=w336) -> ("error out"=w345:errorcluster)
        n107 = call <vilib>:"Simple Error Handler.vi"("error in (no error)"=w345) -> ("error out"=w343:errorcluster)  [unwired: 4 in, 4 out]
        n108 = call "IMAQ Dispose"("error in (no error)"=w343) -> ("error out"=w342:errorcluster)  [unwired: 5 in]
        n109 = local write "Initialized"(FALSE ("Initialized")) -> ()
      }
    }
  }
  "error out" <- w5
  "DMA Words per Image" <- w4
  "Num Frames read" <- w3
  "Image Acquired" <- w2
  "Frames To Acquire" <- w1
